vi "Write Serialization Binder.vi"(8 "error in (no error)":errorcluster, 10 "Serialization Binder":refnum<class "Serialization Binder.lvclass">, 11 "Flatten To JSON Object in":refnum<class "Flatten To JSON Object.lvclass">) -> (0 "error out":errorcluster, 3 "Flatten To JSON Object out":refnum<class "Flatten To JSON Object.lvclass">)   [LabVIEW 2017, in "Flatten To JSON Object.lvclass"]
doc: "Writes the serialization binder."
uses:
  Flatten To JSON Object.lvclass
  Serialization Binder/Serialization Binder.lvclass
  Flatten To JSON Object.lvclass/Flatten To JSON Object.ctl
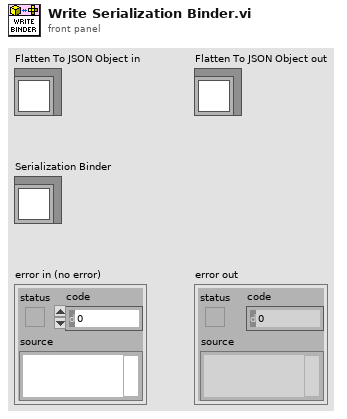
[diagram p1: front panel]
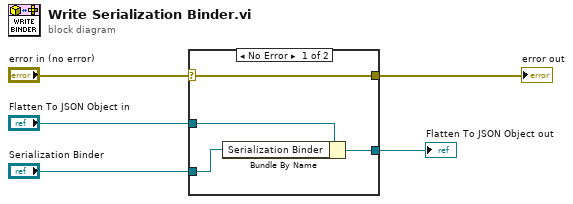
[diagram p0: block diagram]
diagram:
  n1 = case shown="No Error" "error in (no error)" {
    selector: "error in (no error)" -> [w9 w10]
    tunnel: [w9 w10] -> w4
    tunnel: [w7 w11] -> w2
    tunnel: "Flatten To JSON Object in" -> [w8 w11]
    tunnel: "Serialization Binder" -> [w6 _]
    frame No Error {
      n2 = Bundle By Name(cluster=w8, "Serialization Binder"=w6) -> (w7:refnum<class "Flatten To JSON Object.lvclass">)
    }
    frame Error {
    }
  }
  "error out" <- w4
  "Flatten To JSON Object out" <- w2
